vi "Insert Image (Greyscale with Mask).vi"(6 "Greyscale Image Mask in":T1, 7 "Offset (Default: 0,0)":T2, 8 "error in (no error)":errorcluster, 9 "Greyscale Image Destination in":T1, 10 "Greyscale Image Child in":T1, 11 "Greyscale Image Parent in":T1) -> (0 "error out":errorcluster, 3 "Greyscale Image Destination":T1)   [LabVIEW 2020, in "image.lvlib"]
doc: "Copy the pixels from the Child Image where the Mask has non-zero values over the Parent Image with the given offset."
uses:
  image.lvlib
  Greyscale Image.ctl
  common/Image Point (Integer).ctl
  5e3288c8-ee88-4cfe-89cf-31ceca475f5a.vi
  <vilib>/Utility/error.llb/Error Cluster From Error Code.vi
  common/common.lvlib
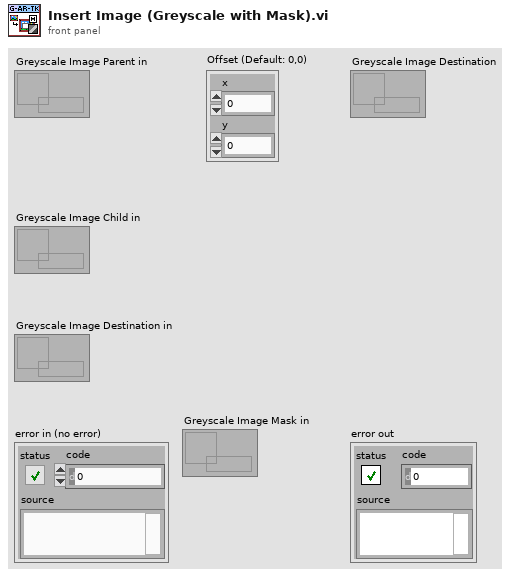
[diagram p1: front panel]
types:
  T1 = typedef "image.lvlib/Greyscale Image.ctl" = refnum<data-value>
  T2 = typedef "common.lvlib/Image Point (Integer).ctl" = cluster{"x":i32, "y":i32}
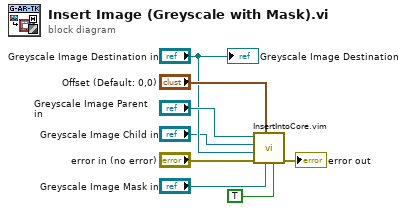
[diagram p0: block diagram]
diagram:
  n1 = call "InsertIntoCore.vim"("Has Mask"=TRUE, "Mask"="Greyscale Image Mask in", "Offset"="Offset (Default: 0,0)", "error in (no error)"="error in (no error)", "Dst"="Greyscale Image Destination in", "Src_Child"="Greyscale Image Child in", "Src_Parent"="Greyscale Image Parent in") -> ("error out"=→"error out":errorcluster)  [unwired: 4 in]
  "Greyscale Image Destination" <- "Greyscale Image Destination in"
